vi "Write All Port Info.vi"(8 "error in (no error)":errorcluster, 10 "Port":T2={"Type"=enum."Serial (VISA)", "Serial Port"="", "IP Address"="0.0.0.0"}, 11 "Data in":refnum<class "Data.lvclass">) -> (0 "error out":errorcluster, 3 "Data out":refnum<class "Data.lvclass">)   [LabVIEW 2018, in "HW Interaction.lvlib" / "Data.lvclass"]
uses:
  Data.lvclass
  Public API/Typedefs/CTL_Port_connection_type.ctl
  Data.lvclass/Data.ctl
  HW Interaction.lvlib
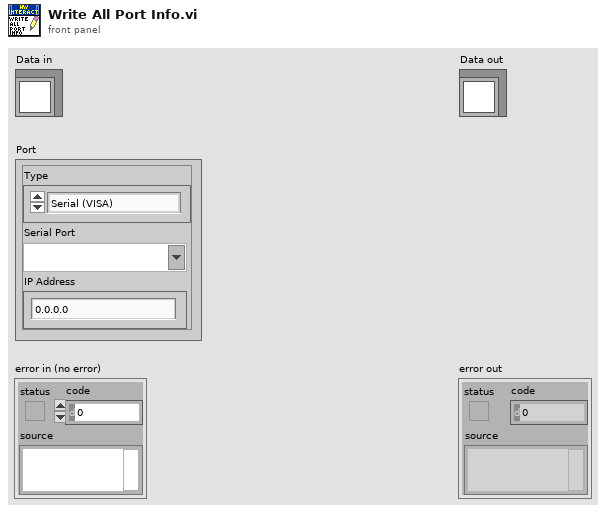
[diagram p1: front panel]
types:
  T1 = typedef "HW Interaction.lvlib/CTL_Port_connection_type.ctl" = enum16{"Serial (VISA)", "TCP/IP"}
  T2 = cluster{"Type":T1, "Serial Port":refnum<visa-resource-name>, "IP Address":string}
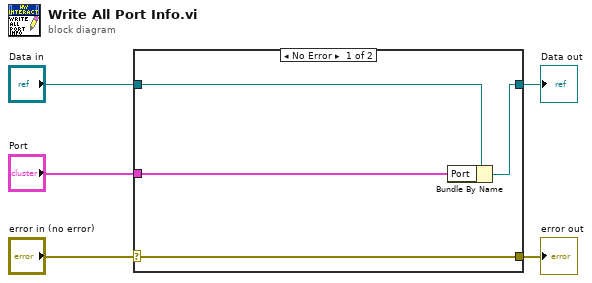
[diagram p0: block diagram]
diagram:
  n1 = case shown="No Error" "error in (no error)" {
    selector: "error in (no error)" -> [w9 w10]
    tunnel: [w9 w10] -> w4
    tunnel: [w7 w11] -> w2
    tunnel: "Data in" -> [w8 w11]
    tunnel: "Port" -> [w6 _]
    frame No Error {
      n2 = Bundle By Name(cluster=w8, "Port"=w6) -> (w7:refnum<class "Data.lvclass">)
    }
    frame Error {
    }
  }
  "error out" <- w4
  "Data out" <- w2
